vi "Reload Display Tables.vi"(8 "Error In":errorcluster, 10 "CD Settings In":T1={"CD Task Dependency"=18446744073709551615, "CD Task Dependency Ref"=18446744073709551615, "CD Task Available Wfms"=[], "CD Task Selected Wfms"=[], "Buffer Length (samples)"=0, "Min Enabled"=FALSE, "Max Enabled "=FALSE, "SP Enabled"=FALSE, "RMS Enabled"=FALSE, "Buffer Length (s)"=0.0, "Task Rate"=0.0, "Number of DAQ Chanels"=0} {"CD Task Dependency Ref" format="%.0x"; "CD Task Dependency" format="%.0x"}, 11 "UI Refs In":T3) -> (0 "Error Out":errorcluster)   [LabVIEW 2017, in "Waveform-Processing-Custom-Device System Explorer.lvlib"]
doc: "This application uses the Referenced obtained from the UI Refs In to reload the channel names back into the displays."
uses:
  Waveform-Processing-Custom-Device System Explorer.lvlib
  Types/UI Refs Ctl.ctl
  Shared/Custom Device Settings.ctl
  <vilib>/NI Veristand/Custom Device API/Custom Device Item Ref.ctl
  Types/State.ctl
  Shared/Waveform-Processing-Custom-Device Shared.lvlib
  <vilib>/NI VeriStand/Custom Device API/Custom Device API.lvlib
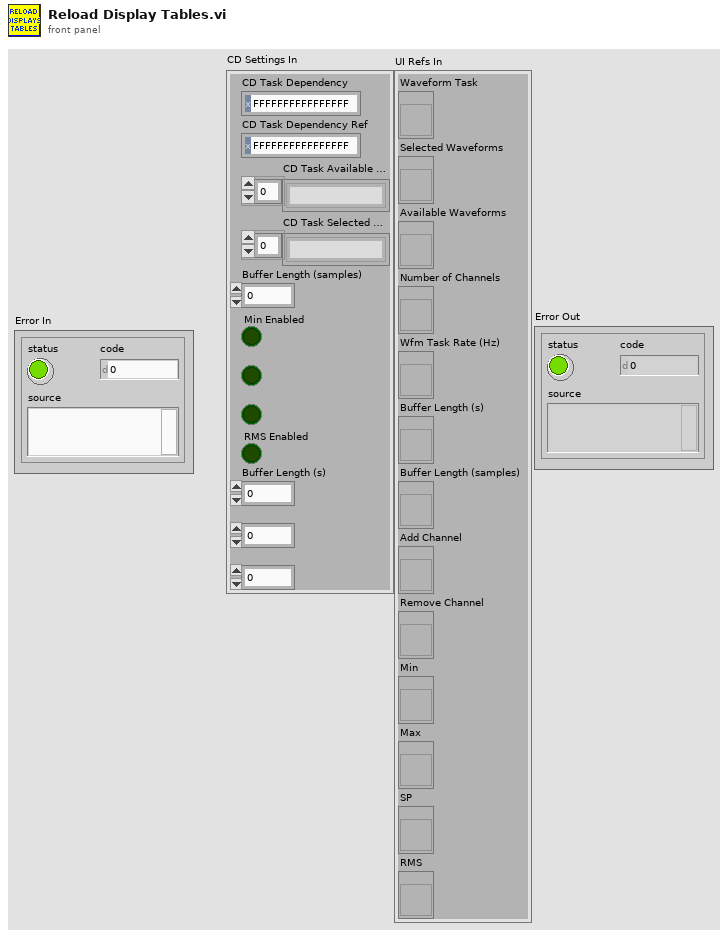
[diagram p1: front panel]
types:
  T1 = typedef "Waveform-Processing-Custom-Device Shared.lvlib/Custom Device Settings.ctl" = cluster{"CD Task Dependency":T2, "CD Task Dependency Ref":T2, "CD Task Available Wfms":string[], "CD Task Selected Wfms":string[], "Buffer Length (samples)":u32, "Min Enabled":bool, "Max Enabled ":bool, "SP Enabled":bool, "RMS Enabled":bool, "Buffer Length (s)":dbl, "Task Rate":dbl, "Number of DAQ Chanels":u32}
  T2 = typedef "Custom Device API.lvlib/Custom Device Item Ref.ctl" = u64
  T3 = typedef "Waveform-Processing-Custom-Device Shared.lvlib/UI Refs Ctl.ctl" = cluster{"Waveform Task":refnum<vi>, "Selected Waveforms":refnum<vi>, "Available Waveforms":refnum<vi>, "Number of Channels":refnum<vi>, "Wfm Task Rate (Hz)":refnum<vi>, "Buffer Length (s)":refnum<vi>, "Buffer Length (samples)":refnum<vi>, "Add Channel":refnum<vi>, "Remove Channel":refnum<vi>, "Min":refnum<vi>, "Max":refnum<vi>, "SP":refnum<vi>, "RMS":refnum<vi>}
  T4 = typedef "Waveform-Processing-Custom-Device System Explorer.lvlib/State.ctl" = enum16{"Start", "1", "2", "3", "4", "5", "6", "7", "8", "9", "End"}
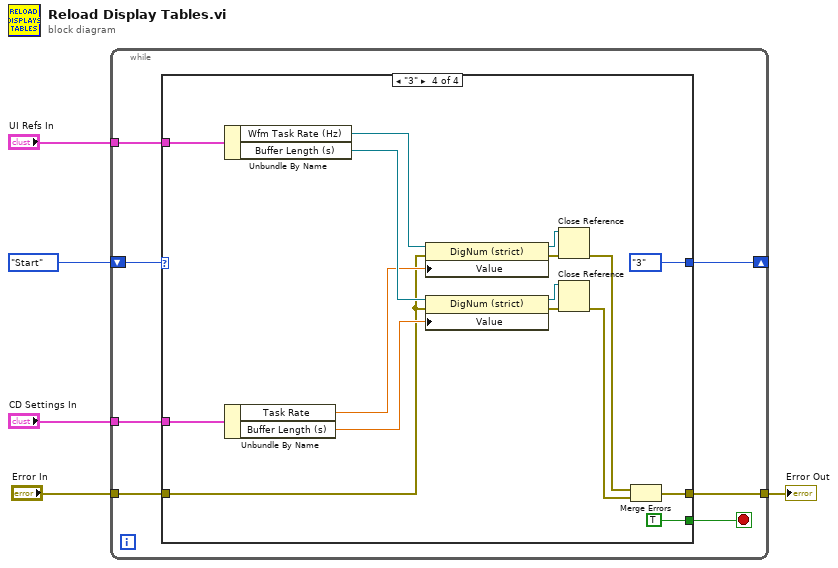
[diagram p0: block diagram]
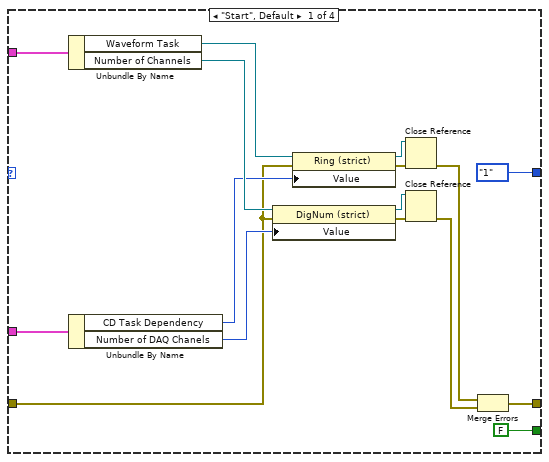
[diagram p2: hidden frame]
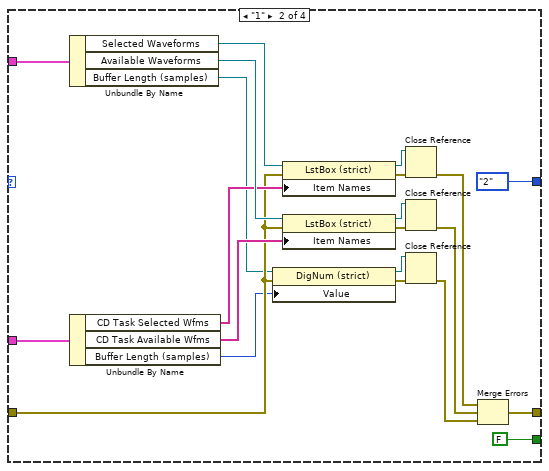
[diagram p3: hidden frame]
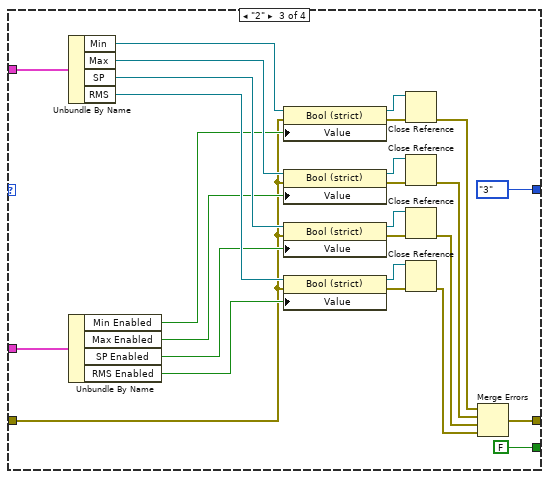
[diagram p4: hidden frame]
diagram:
  n1 = while {
    shift-right: [w11] -> _
    shift-left: State."Start" ("Enum") -> [w12]
    tunnel: "UI Refs In" -> [w10]
    tunnel: "CD Settings In" -> [w9]
    tunnel: "Error In" -> [w8]
    tunnel: [w7] -> w1
    stop <- w6 stop-if-true
    n2 = case shown="\"3\"" w12 {
      tunnel: [State."1" ("Enum") State."2" ("Enum") State."3" ("Enum") State."3" ("Enum")] -> w11
      tunnel: w10 -> [w23 w44 w66 w86]
      tunnel: w9 -> [w22 w43 w65 w85]
      tunnel: w8 -> [w17 w34 w56 w80]
      tunnel: [w15 w37 w54 w78] -> w7
      tunnel: [FALSE FALSE FALSE TRUE] -> w6
      frame "Start", Default {
        n3 = Unbundle By Name(w23) -> ("Waveform Task"=w20:refnum<vi>, "Number of Channels"=w21:refnum<vi>)
        n4 = Unbundle By Name(w22) -> ("CD Task Dependency"=w19:T2, "Number of DAQ Chanels"=w18:u32)
        n5 = property class="DigNum (strict)"(reference=w21, error in=w17, "Value"=w18) -> (reference out=w26:refnum<vi>, error out=w25:errorcluster)
        n6 = property class="Ring (strict)"(reference=w20, error in=w17, "Value"=w19) -> (reference out=w27:refnum<vi>, error out=w28:errorcluster)
        n7 = Close Reference(reference=w27, error in (no error)=w28) -> (error out=w13:errorcluster)
        n8 = Close Reference(reference=w26, error in (no error)=w25) -> (error out=w14:errorcluster)
        n9 = Merge Errors(w13, w14) -> (w15:errorcluster)
      }
      frame "1" {
        n10 = Unbundle By Name(w44) -> ("Selected Waveforms"=w41:refnum<vi>, "Available Waveforms"=w42:refnum<vi>, "Buffer Length (samples)"=w30:refnum<vi>)
        n11 = Unbundle By Name(w43) -> ("CD Task Selected Wfms"=w40:string[], "CD Task Available Wfms"=w39:string[], "Buffer Length (samples)"=w29:u32)
        n12 = property class="DigNum (strict)"(reference=w30, error in=w34, "Value"=w29) -> (reference out=w31:refnum<vi>, error out=w32:errorcluster)
        n13 = property class="LstBox (strict)"(reference=w41, error in=w34, "Item Names"=w40) -> (reference out=w48:refnum<vi>, error out=w49:errorcluster)
        n14 = property class="LstBox (strict)"(reference=w42, error in=w34, "Item Names"=w39) -> (reference out=w47:refnum<vi>, error out=w46:errorcluster)
        n15 = Close Reference(reference=w48, error in (no error)=w49) -> (error out=w35:errorcluster)
        n16 = Close Reference(reference=w47, error in (no error)=w46) -> (error out=w36:errorcluster)
        n17 = Close Reference(reference=w31, error in (no error)=w32) -> (error out=w33:errorcluster)
        n18 = Merge Errors(w35, w36, w33) -> (w37:errorcluster)
      }
      frame "2" {
        n19 = Unbundle By Name(w66) -> ("Min"=w61:refnum<vi>, "Max"=w62:refnum<vi>, "SP"=w63:refnum<vi>, "RMS"=w64:refnum<vi>)
        n20 = Unbundle By Name(w65) -> ("Min Enabled"=w60:bool, "Max Enabled"=w59:bool, "SP Enabled"=w58:bool, "RMS Enabled"=w57:bool)
        n21 = property class="Bool (strict)"(reference=w61, error in=w56, "Value"=w60) -> (reference out=w70:refnum<vi>, error out=w71:errorcluster)
        n22 = property class="Bool (strict)"(reference=w62, error in=w56, "Value"=w59) -> (reference out=w74:refnum<vi>, error out=w75:errorcluster)
        n23 = property class="Bool (strict)"(reference=w63, error in=w56, "Value"=w58) -> (reference out=w73:refnum<vi>, error out=w72:errorcluster)
        n24 = property class="Bool (strict)"(reference=w64, error in=w56, "Value"=w57) -> (reference out=w69:refnum<vi>, error out=w68:errorcluster)
        n25 = Close Reference(reference=w70, error in (no error)=w71) -> (error out=w50:errorcluster)
        n26 = Close Reference(reference=w74, error in (no error)=w75) -> (error out=w51:errorcluster)
        n27 = Close Reference(reference=w73, error in (no error)=w72) -> (error out=w52:errorcluster)
        n28 = Close Reference(reference=w69, error in (no error)=w68) -> (error out=w53:errorcluster)
        n29 = Merge Errors(w50, w51, w52, w53) -> (w54:errorcluster)
      }
      frame "3" {
        n30 = Unbundle By Name(w86) -> ("Wfm Task Rate (Hz)"=w83:refnum<vi>, "Buffer Length (s)"=w84:refnum<vi>)
        n31 = Unbundle By Name(w85) -> ("Task Rate"=w82:dbl, "Buffer Length (s)"=w81:dbl)
        n32 = property class="DigNum (strict)"(reference=w83, error in=w80, "Value"=w82) -> (reference out=w90:refnum<vi>, error out=w91:errorcluster)
        n33 = property class="DigNum (strict)"(reference=w84, error in=w80, "Value"=w81) -> (reference out=w89:refnum<vi>, error out=w88:errorcluster)
        n34 = Close Reference(reference=w90, error in (no error)=w91) -> (error out=w76:errorcluster)
        n35 = Close Reference(reference=w89, error in (no error)=w88) -> (error out=w77:errorcluster)
        n36 = Merge Errors(w76, w77) -> (w78:errorcluster)
      }
    }
  }
  "Error Out" <- w1
